vi "Reset_db_for_cache_waveforms.vi"() -> ()   [LabVIEW 2013]
uses:
  <vilib>/addons/database/Connection.llb/Conn Execute.vi
  <vilib>/addons/database/Recordset.llb/Rec Destroy - Connection.vi
  <vilib>/addons/database/NI_Database_API.lvlib
panel:
  out "Query String":string
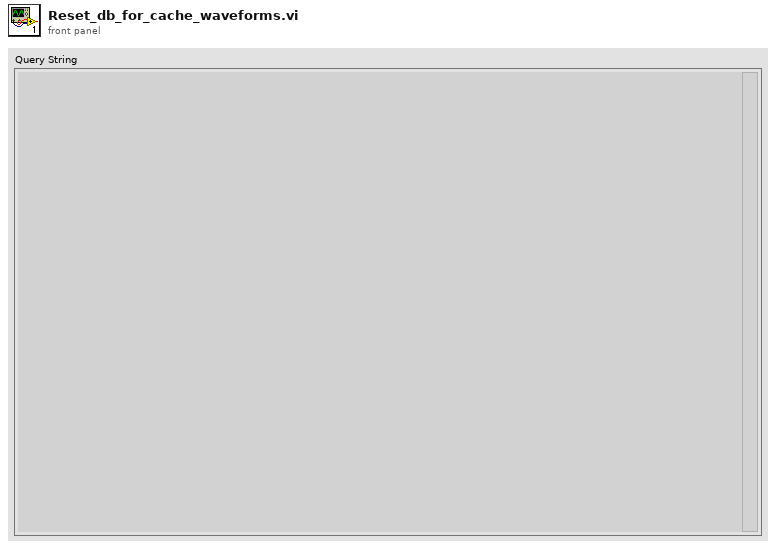
[diagram p1: front panel]
types:
  T1 = typedef "NI_Database_API.lvlib/Conn ObjectReference.ctl" = refnum<k1>
  T2 = typedef "NI_Database_API.lvlib/Rec ObjectReference.ctl" = refnum<k1>
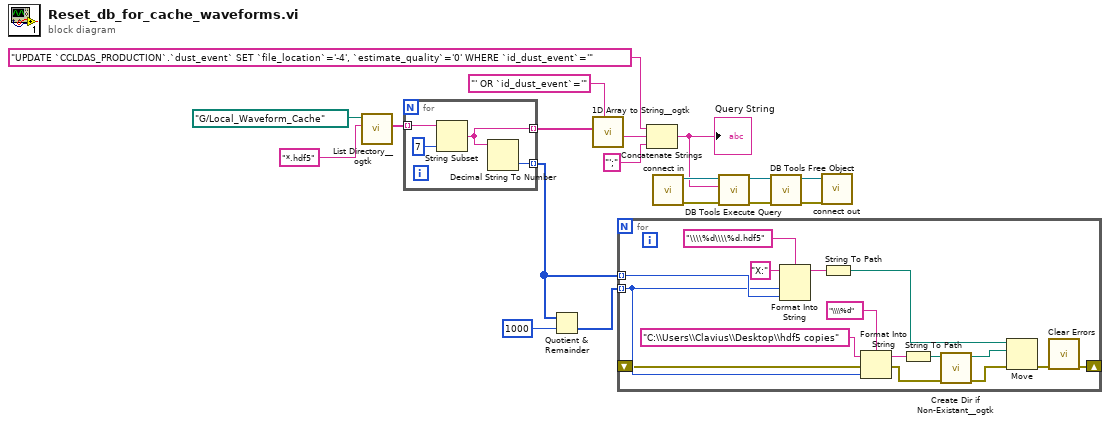
[diagram p0: block diagram]
diagram:
  n1 = call <userlib>:"List Directory__ogtk.vi"("pattern"="*.hdf5", "directory path"=path "G:/Local_Waveform_Cache") -> ("file names"=w18:string[])  [unwired: 2 in, 3 out]
  n2 = for {
    tunnel: w18 -> [w22] mode=indexing
    tunnel: [w20] -> w16 mode=indexing
    tunnel: [w19] -> w9 mode=indexing
    n3 = String Subset(string=w22, length (rest)=7 ("length (rest)")) -> (substring=w20:string)  [unwired: 1 in]
    n4 = Decimal String To Number(string=w20) -> (number=w19:i32)  [unwired: 2 in, 1 out]
  }
  n5 = Quotient & Remainder(x=w9, y=1000) -> (floor(x/y)=w10:i32[])  [unwired: 1 out]
  n6 = call <userlib>:"1D Array to String__ogtk.vi"("delimiter (Tab)"="' OR `id_dust_event`='", "Array of Strings"=w16) -> ("delimited string"=w14:string)  [unwired: 9 in]
  n7 = for {
    tunnel: w10 -> [w30] mode=indexing
    tunnel: w9 -> [w31] mode=indexing
    shift-right: [w24] -> _
    shift-left: _ -> [w23]
    n8 = Format Into String(format string="\\\\%d\\\\%d.hdf5", initial string="X:", w30, w31) -> (resulting string=w38:string)  [unwired: 1 in, 1 out]
    n9 = String To Path(string=w38) -> (path=w37:path)
    n10 = Format Into String(format string="\\\\%d", initial string="C:\\Users\\Clavius\\Desktop\\hdf5 copies", error in=w23, w30) -> (resulting string=w34:string, error out=w27:errorcluster)
    n11 = String To Path(string=w34) -> (path=w36:path)
    n12 = call <userlib>:"Create Dir if Non-Existant__ogtk.vi"("error in (no error)"=w27, "Directory Path"=w36) -> ("error out"=w26:errorcluster, "dup Directory Path"=w29:path)  [unwired: 7 in, 1 out]
    n13 = Move(source path=w37, error in=w26, 10:w29) -> (error out=w25:errorcluster)  [unwired: 2 in, 2 out]
    n14 = call <vilib>:"Clear Errors.vi"("error in (no error)"=w25) -> ("error out"=w24:errorcluster)  [unwired: 6 in]
  }
  n15 = Concatenate Strings("UPDATE `CCLDAS_PRODUCTION`.`dust_event` SET `file_location`='-4', `estimate_quality`='0' WHERE `id_dust_event`='" ("string"), w14, "';" ("string")) -> (w2:string)
  "Query String" <- w2
  n16 = call "connect in.vi"() -> ("error out"=w5:errorcluster, "Database Connection"=w6:T1)  [unwired: 7 in, 1 out]
  n17 = call-poly <vilib>:"DB Tools Execute Query.vi"("error in (no error)"=w5, "SQL query"=w2, "connection reference"=w6) -> ("error out"=w3:errorcluster, "recordset reference"=w4:T2)  [unwired: 5 in]
  n18 = call-poly <vilib>:"DB Tools Free Object.vi"("error in (no error)"=w3, "recordset reference"=w4) -> ("error out"=w7:errorcluster, "connection reference"=w8:T1)  [unwired: 8 in]
  n19 = call "connect out.vi"("error in (no error)"=w7, "connection reference"=w8) -> ()  [unwired: 9 in, 1 out]
